vi "Play.vi"(0 "Universal Robot.lvclass in":refnum<class "Universal Robot.lvclass">, 5 "error in (no error)":errorcluster) -> (14 "Universal Robot.lvclass out":refnum<class "Universal Robot.lvclass">, 19 "error out":errorcluster)   [LabVIEW 2016, in "Universal Robot.lvclass"]
uses:
  Universal Robot.lvclass
  Universal Robot.lvclass/Universal Robot.ctl
  DashboardServer/Dashboard Server.lvclass
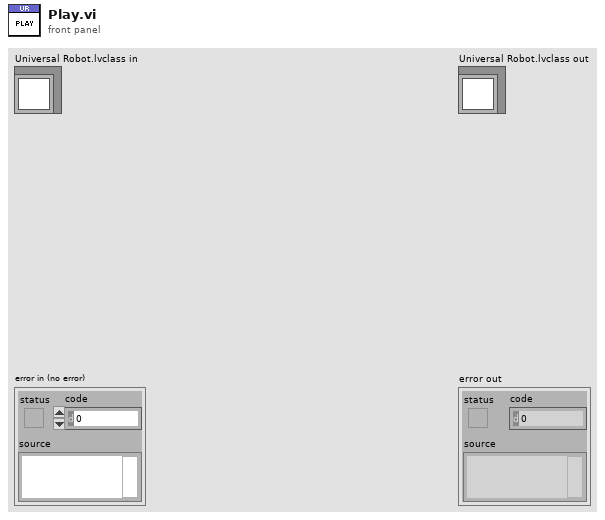
[diagram p1: front panel]
types:
  T1 = typedef "Universal Robot.lvclass/RobotStatus.ctl" = cluster{"Robot Mode":T2, "Operational Mode":T3, "Safety Status":T4, "Remote Control":bool}
  T2 = typedef "Universal Robot.lvclass/RobotMode.ctl" = enum16{"INVALID", "NO_CONTROLLER", "DISCONNECTED", "CONFIRM_SAFETY", "BOOTING", "POWER_OFF", "POWER_ON", "IDLE", "BACKDRIVE", "RUNNING"}
  T3 = typedef "Universal Robot.lvclass/OperationalMode.ctl" = enum16{"NONE", "MANUAL", "AUTOMATIC"}
  T4 = typedef "Universal Robot.lvclass/SafetyStatus.ctl" = enum16{"INVALID", "NORMAL", "REDUCED", "PROTECTIVE_STOP", "RECOVERY", "SAFEGAURD_STOP", "SYSTEM_EMERGENCY_STOP", "ROBOT_EMERGENCY_STOP", "VIOLATION", "FAULT", "AUTOMATIC_MODE_SAFEGAURD_STOP", "SYSTEM_THREE_POSITION_ENABLING_STOP"}
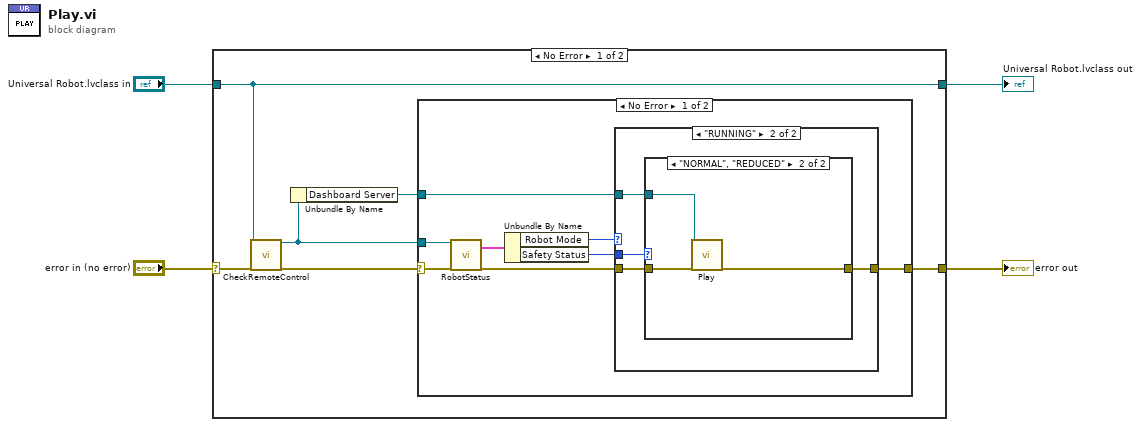
[diagram p0: block diagram]
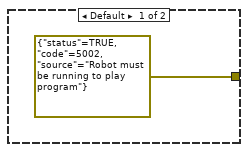
[diagram p2: hidden frame]
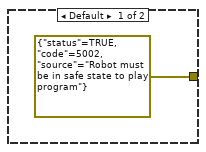
[diagram p3: hidden frame]
diagram:
  n1 = case shown="No Error" "error in (no error)" {
    selector: "error in (no error)" -> [w9 w30]
    tunnel: [w10 w30] -> w3
    tunnel: "Universal Robot.lvclass in" -> [w8 w29]
    tunnel: [w8 w29] -> w1
    frame No Error {
      n2 = call-dynamic "CheckRemoteControl.vi"("Universal Robot.lvclass in"=w8, "error in (no error)"=w9) -> ("Universal Robot.lvclass out"=w5:refnum<class "Universal Robot.lvclass">, "error out"=w6:errorcluster)  [unwired: 16 in]
      n3 = Unbundle By Name(w5) -> ("Dashboard Server"=w7:refnum<class "Dashboard Server.lvclass">)
      n4 = case shown="No Error" w6 {
        selector: w6 -> [w17 w28]
        tunnel: [w18 w28] -> w10
        tunnel: w7 -> [w12 _]
        tunnel: w5 -> [w16 _]
        frame No Error {
          n5 = call-dynamic "RobotStatus.vi"("Universal Robot.lvclass in"=w16, "error in (no error)"=w17) -> ("Robot Status"=w15:T1, "error out"=w14:errorcluster)  [unwired: 15 in, 1 out]
          n6 = Unbundle By Name(w15) -> ("Robot Mode"=w13:T2, "Safety Status"=w11:T4)
          n7 = case shown="\"RUNNING\"" w13 {
            tunnel: [errorcluster {"status"=TRUE, "code"=5002, "source"="Robot must be running to play program"} ("error out") w22] -> w18
            tunnel: w14 -> [_ w23]
            tunnel: w12 -> [_ w21]
            tunnel: w11 -> [_ w20]
            frame Default {
            }
            frame "RUNNING" {
              n8 = case shown="\"NORMAL\", \"REDUCED\"" w20 {
                tunnel: w23 -> [_ w27]
                tunnel: [errorcluster {"status"=TRUE, "code"=5002, "source"="Robot must be in safe state to play program"} ("error out") w25] -> w22
                tunnel: w21 -> [_ w26]
                frame Default {
                }
                frame "NORMAL", "REDUCED" {
                  n9 = call-dynamic "Play.vi"("DashboardServer in"=w26, "error in (no error)"=w27) -> ("error out"=w25:errorcluster)  [unwired: 16 in, 1 out]
                }
              }
            }
          }
        }
        frame Error {
        }
      }
    }
    frame Error {
    }
  }
  "error out" <- w3
  "Universal Robot.lvclass out" <- w1
